vi "OnInitMenu.vi"(8 "error in (no error)":errorcluster, 11 "Game in":refnum<class "Game.lvclass">) -> (0 "error out":errorcluster, 3 "Game out":refnum<class "Game.lvclass">)   [LabVIEW 2019, in "RT_Game.lvlib" / "Game.lvclass"]
uses:
  Game.lvclass
  SpritesCluster.ctl
  RT_Sprite/RT_Sprite.lvclass
  C:/Users/FreshBob/Dropbox/VIs/myRIO_GameConsole/RT/RT_Game/GameObject/GameObject.lvclass
  Coordinate.ctl
  Game.lvclass/Game.ctl
  GameMenu/GameMenu.lvclass/GameMenu.ctl
  GameMenu/Read Position.vi
  GameMenu/GameMenu.lvclass
  Highscore/Highscore.lvclass
  GameObject/GameObject.lvclass
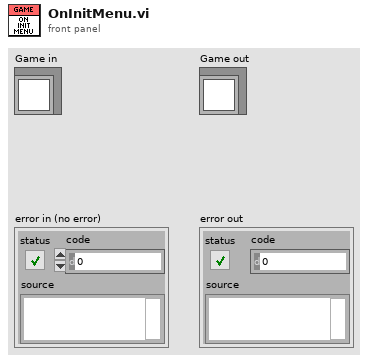
[diagram p1: front panel]
types:
  T1 = typedef "RT_Game.lvlib/Game.lvclass/Coordinate.ctl" = cluster{"x":dbl, "y":dbl}
  T2 = typedef "RT_Game.lvlib/Game.lvclass/SpritesCluster.ctl" = cluster{"Sprite1":refnum<class "RT_Sprite.lvclass">, "Sprite2":refnum<class "RT_Sprite.lvclass">, "Sprite3":refnum<class "RT_Sprite.lvclass">}
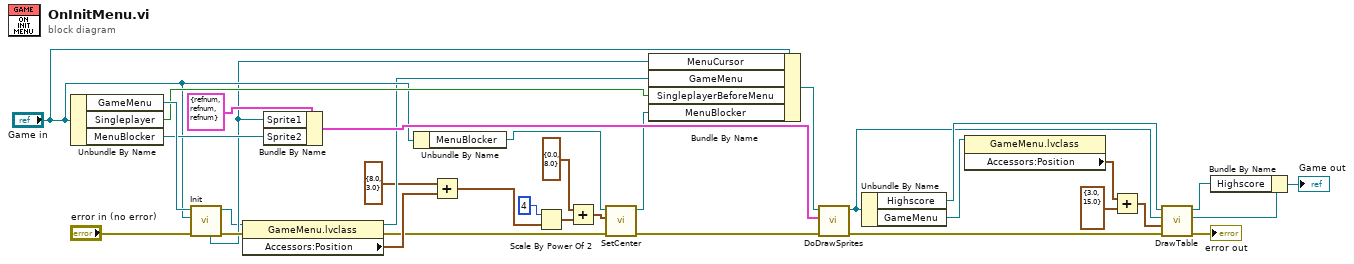
[diagram p0: block diagram]
diagram:
  n1 = Unbundle By Name("Game in") -> ("GameMenu"=w28:refnum<class "GameMenu.lvclass">, "Singleplayer"=w27:bool, "MenuBlocker"=w16:refnum<class "RT_Sprite.lvclass">)
  n2 = call "Init.vi"("error in (no error)"="error in (no error)", "Game (readonly)"="Game in", "GameMenu in"=w28) -> ("error out"=w30:errorcluster, "GameMenu out"=w13:refnum<class "GameMenu.lvclass">, "CursorSprite"=w14:refnum<class "RT_Sprite.lvclass">)  [unwired: 6 in]
  n3 = property class="GameMenu.lvclass"(reference=w13, error in=w30) -> (reference out=w12:refnum<class "GameMenu.lvclass">, error out=w2:errorcluster, "Accessors:Position"=w8:T1)
  n4 = Bundle By Name(cluster=T2 {"Sprite1"=refnum, "Sprite2"=refnum, "Sprite3"=refnum} ("Sprites in"), "Sprite1"=w14, "Sprite2"=w16) -> (w34:T2)
  n5 = Unbundle By Name("Game in") -> ("MenuBlocker"=w10:refnum<class "RT_Sprite.lvclass">)
  n6 = Add(x=T1 {"x"=8.0, "y"=3.0}, y=w8) -> (x+y=w7:T1)
  n7 = Scale By Power Of 2(n=i16 4, x=w7) -> (x*2^n=w3:T1)
  n8 = Add(x=T1 {"x"=0.0, "y"=8.0}, y=w3) -> (x+y=w1:T1)
  n9 = call "SetCenter.vi"("error in (no error)"=w2, "center_position"=w1, "GameObject in"=w10) -> ("error out"=w11:errorcluster, "GameObject out"=w9:refnum<class "RT_Sprite.lvclass">)  [unwired: 7 in]
  n10 = Bundle By Name(cluster="Game in", "MenuCursor"=w14, "GameMenu"=w12, "SingleplayerBeforeMenu"=w27, "MenuBlocker"=w9) -> (w32:refnum<class "Game.lvclass">)
  n11 = call "DoDrawSprites.vi"("error in (no error)"=w11, "Sprites in"=w34, "Game in"=w32) -> ("error out"=w31:errorcluster, "Game out"=w22:refnum<class "Game.lvclass">)  [unwired: 6 in, 1 out]
  n12 = Unbundle By Name(w22) -> ("Highscore"=w24:refnum<class "Highscore.lvclass">, "GameMenu"=w18:refnum<class "GameMenu.lvclass">)
  n13 = property class="GameMenu.lvclass"(reference=w18) -> ("Accessors:Position"=w17:T1)  [unwired: 1 in, 2 out]
  n14 = Add(x=w17, y=T1 {"x"=3.0, "y"=15.0} ("Position")) -> (x+y=w19:T1)
  n15 = call "DrawTable.vi"("error in (no error)"=w31, "Position"=w19, "GameIn"=w22, "Highscore in"=w24) -> ("error out"=→"error out":errorcluster, "GameOut"=w21:refnum<class "Game.lvclass">, "Highscore out"=w23:refnum<class "Highscore.lvclass">)  [unwired: 5 in]
  n16 = Bundle By Name(cluster=w21, "Highscore"=w23) -> (→"Game out":refnum<class "Game.lvclass">)
